vi "RIOduino Periodic.vi"() -> ()   [LabVIEW 2014]
uses:
  <vilib>/Rock Robotics/SystemInterfaces/Typedef/FPGA_TypedefDigitalModule.ctl
  <vilib>/Rock Robotics/SystemInterfaces/i2clib/i2c_bus.ctl
  General_VI/Global Var.vi
panel:
  in  "y":dbl=5.0
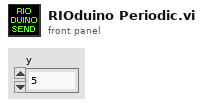
[diagram p1: front panel]
types:
  T1 = typedef "WPI_DriverStationRobotMode2.ctl" = enum16{"Autonomous Disabled", "Autonomous Enabled", "Teleop Disabled", "Teleop Enabled", "Disconnected", "Finish", "Test Disabled", "Test Enabled", "Emergency Stopped"}
  T2 = typedef "WPI_DriverStationAllianceInfo.ctl" = enum16{"Red", "Blue", "Invalid"}
  T3 = typedef "WPI_I2CDevRef.ctl" = cluster{"DevStatus":errorcluster, "Controller":T4, "Device Address":u8, "Handle":i32, "I2C Bus":T5}
  T4 = typedef "FPGA_TypedefDigitalModule.ctl" = enum16{"Controller 1"}
  T5 = typedef "i2c_bus.ctl" = enum16{"I2C On-Board", "I2C MXP", "Invalid"}
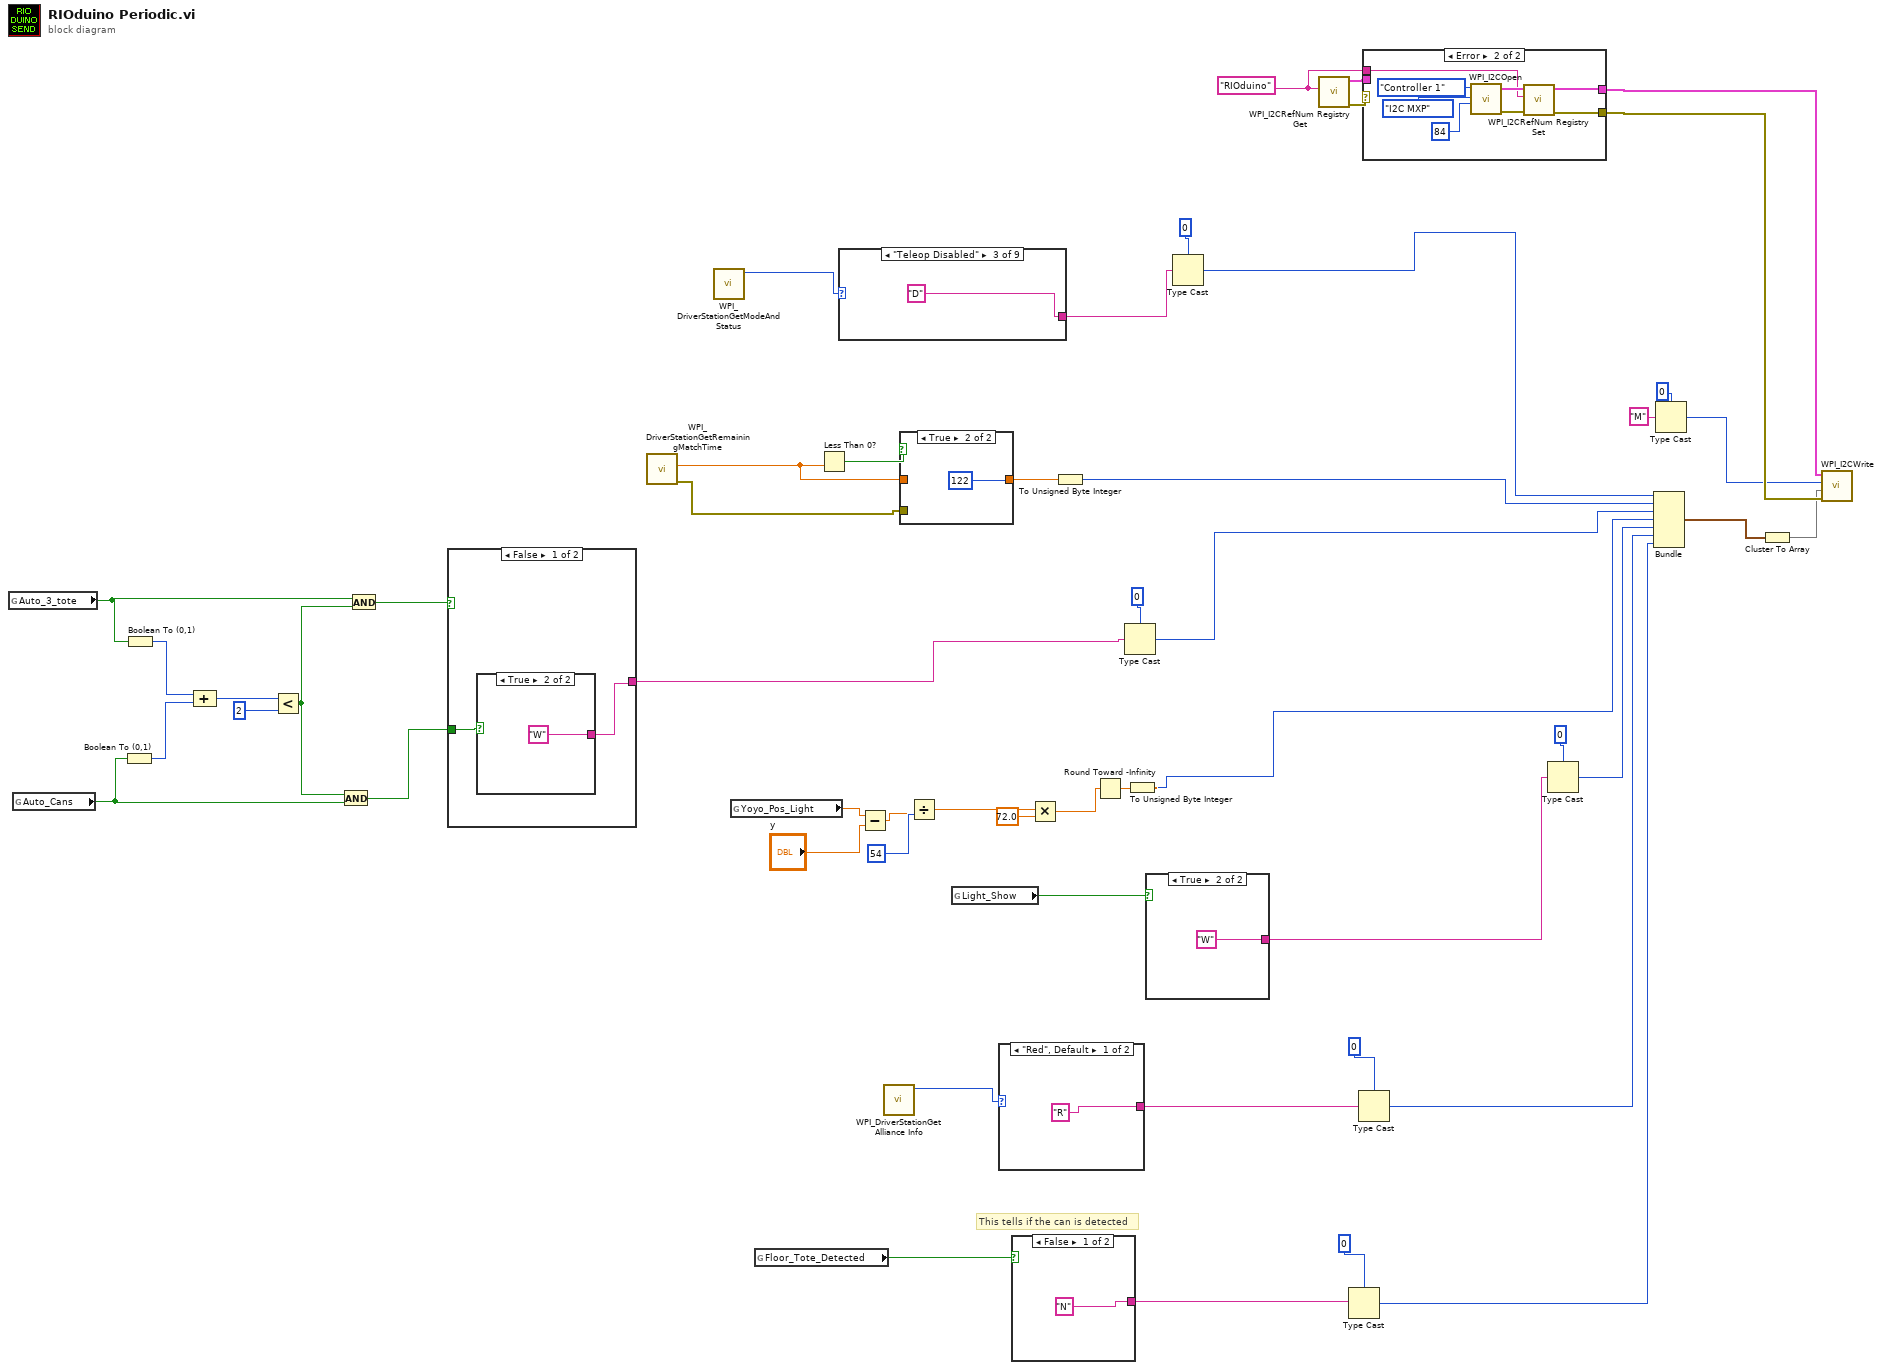
[diagram p0: block diagram]
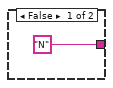
[diagram p2: hidden frame]
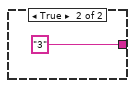
[diagram p3: hidden frame]
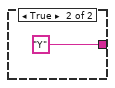
[diagram p4: hidden frame]
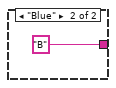
[diagram p5: hidden frame]
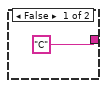
[diagram p6: hidden frame]
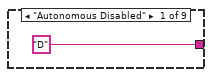
[diagram p8: hidden frame]
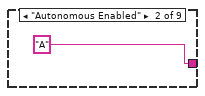
[diagram p9: hidden frame]
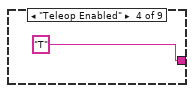
[diagram p10: hidden frame]
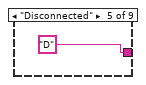
[diagram p11: hidden frame]
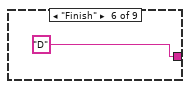
[diagram p12: hidden frame]
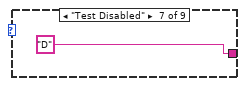
[diagram p13: hidden frame]
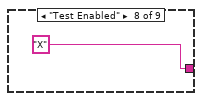
[diagram p14: hidden frame]
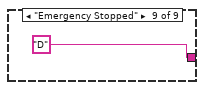
[diagram p15: hidden frame]
diagram:
  w50 = "RIOduino" ("refnum name")
  # "This tells if the can is detected"
  n1 = global read "Global Var.vi" "Auto_3_tote"() -> (w6:bool)
  n2 = global read "Global Var.vi" "Auto_Cans"() -> (w7:bool)
  n3 = Boolean To (0,1)(Boolean=w7) -> (0, 1=w9:i16)
  n4 = Boolean To (0,1)(Boolean=w6) -> (0, 1=w10:i16)
  n5 = Compound Arithmetic op=ADD(w10, w9) -> (w8:i16)
  n6 = Less?(x=w8, y=i16 2) -> (x < y?=w5:bool)
  n7 = And(x=w5, y=w7) -> (x .and. y?=w3:bool)
  n8 = And(x=w6, y=w5) -> (x .and. y?=w4:bool)
  n9 = case shown="False" w4 {
    tunnel: w3 -> [w54 _]
    tunnel: [w53 "3"] -> w2
    frame False {
      n10 = case shown="True" w54 {
        tunnel: ["N" "W"] -> w53
        frame False {
        }
        frame True {
        }
      }
    }
    frame True {
    }
  }
  n11 = call <vilib>:"WPI_DriverStationGetRemainingMatchTime.vi"() -> ("error out"=w29:errorcluster, "Match Time(s)"=w1:sgl)  [unwired: 10 in]
  n12 = call <vilib>:"WPI_DriverStationGetModeAndStatus.vi"() -> ("Robot Mode"=w41:T1)  [unwired: 10 in, 1 out]
  n13 = global read "Global Var.vi" "Yoyo_Pos_Light"() -> (w19:dbl)
  n14 = global read "Global Var.vi" "Floor_Tote_Detected"() -> (w15:bool)
  n15 = Less Than 0?(x=w1) -> (x < 0?=w47:bool)
  n16 = case shown="\"Teleop Disabled\"" w41 {
    tunnel: ["D" "A" "D" "T" "D" "D" "D" "X" "D"] -> w32
    frame "Autonomous Disabled" {
    }
    frame "Autonomous Enabled" {
    }
    frame "Teleop Disabled" {
    }
    frame "Teleop Enabled" {
    }
    frame "Disconnected" {
    }
    frame "Finish" {
    }
    frame "Test Disabled" {
    }
    frame "Test Enabled" {
    }
    frame "Emergency Stopped" {
    }
  }
  n17 = Subtract(x=w19, y="y") -> (x-y=w18:dbl)
  n18 = call <vilib>:"WPI_DriverStationGet Alliance Info.vi"() -> ("Alliance"=w27:T2)  [unwired: 10 in, 1 out]
  n19 = case shown="True" w47 {
    tunnel: w1 -> [w67 _]
    tunnel: [w67 122] -> w46
    tunnel: w29 -> [_ _]
    frame False {
    }
    frame True {
    }
  }
  n20 = Divide(x=w18, y=54) -> (x/y=w20:dbl)
  n21 = global read "Global Var.vi" "Light_Show"() -> (w22:bool)
  n22 = case shown="\"Red\", Default" w27 {
    tunnel: ["R" "B"] -> w25
    frame "Red", Default {
    }
    frame "Blue" {
    }
  }
  n23 = case shown="False" w15 {
    tunnel: ["N" "Y"] -> w13
    frame False {
    }
    frame True {
    }
  }
  n24 = Multiply(x=w20, y=72.0) -> (x*y=w16:dbl)
  n25 = To Unsigned Byte Integer(number=w46) -> (unsigned 8bit integer=w40:u8)
  n26 = Round Toward -Infinity(1:w16) -> (0:w45:dbl)
  n27 = Type Cast(type=u8 0, x=w2) -> (*(type *) &x=w34:u8)
  n28 = To Unsigned Byte Integer(number=w45) -> (unsigned 8bit integer=w39:u8)
  n29 = case shown="True" w22 {
    tunnel: ["C" "W"] -> w28
    frame False {
    }
    frame True {
    }
  }
  n30 = Type Cast(type=u8 0, x=w32) -> (*(type *) &x=w31:u8)
  n31 = call <vilib>:"WPI_I2CRefNum Registry Get.vi"("refnum name"=w50) -> ("error out"=w48:errorcluster, "I2CDevRef"=w49:T3)  [unwired: 9 in]
  n32 = Type Cast(type=u8 0, x=w13) -> (*(type *) &x=w12:u8)
  n33 = Type Cast(type=u8 0, x=w25) -> (*(type *) &x=w24:u8)
  n34 = case shown="Error" w48 {
    selector: w48 -> [w76 _]
    tunnel: [w76 w77] -> w52
    tunnel: [w75 w78] -> w51
    tunnel: w49 -> [w75 _]
    tunnel: w50 -> [_ w79]
    frame No Error {
    }
    frame Error {
      n35 = call <vilib>:"WPI_I2COpen.vi"("Device Address"=u8 84, "I2C Bus"=i2c_bus."I2C MXP", "Controller"=FPGA_TypedefDigitalModule."Controller 1") -> ("error out"=w81:errorcluster, "I2CDevRef"=w80:T3)  [unwired: 7 in]
      n36 = call <vilib>:"WPI_I2CRefNum Registry Set.vi"("error in (no error)"=w81, "refnum name"=w79, "I2CDevRef"=w80) -> ("error out"=w77:errorcluster, "I2CDevRef"=w78:T3)  [unwired: 7 in]
    }
  }
  n37 = Type Cast(type=u8 0, x=w28) -> (*(type *) &x=w37:u8)
  n38 = Bundle(w31, w40, w34, w39, w37, w24, w12) -> (w38:cluster{u8, u8, u8, u8, u8, u8, u8})  [unwired: 1 in]
  n39 = Type Cast(type=u8 0, x="M") -> (*(type *) &x=w42:u8)
  n40 = Cluster To Array(cluster=w38) -> (array=w30:u8[])
  n41 = call <vilib>:"WPI_I2CWrite.vi"("error in (no error)"=w52, "I2CDataToSend"=w30, "I2CRegister"=w42, "I2CDevRef"=w51) -> ()  [unwired: 6 in, 2 out]
